vi "bt-send_data.vi"(8 "error in (no error)":errorcluster, 10 "send data (string)":string) -> (0 "error out":errorcluster, 2 "timeout?":bool)   [LabVIEW 2023, in "bt-interface.lvlib"]
uses:
  bt-interface.lvlib
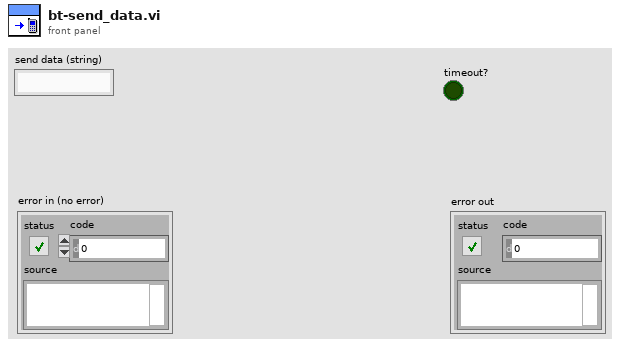
[diagram p1: front panel]
types:
  T1 = enum16{"init", "broadcast_data", "receive_data", "close", "clear_visa"}
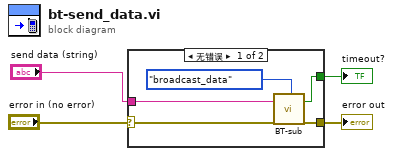
[diagram p0: block diagram]
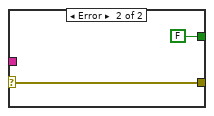
[diagram p2: hidden frame]
diagram:
  n1 = case shown="无错误" "error in (no error)" {
    selector: "error in (no error)" -> [w9 w11]
    tunnel: [w8 w11] -> w3
    tunnel: "send data (string)" -> [w7 _]
    tunnel: [w5 FALSE ("timeout?")] -> w1
    frame No Error {
      n2 = call "BT-sub.vi"("send data"=w7, "error in (no error)"=w9, "mode"=T1."broadcast_data") -> ("timeout?"=w5:bool, "error IO"=w8:errorcluster)  [unwired: 14 in, 1 out]
    }
    frame Error {
    }
  }
  "error out" <- w3
  "timeout?" <- w1
